vi "SRS865A--read--V2.vi"(8 "error in (no error)":errorcluster, 11 "VISA resource name":refnum<visa-resource-name>) -> (0 "error out":errorcluster, 1 "freq out":dbl, 2 "zi out (V)":cdb, 3 "VISA resource name out":refnum<visa-resource-name>)   [LabVIEW 2018]
uses:
  <instrlib>/Stanford Research SR865/Stanford Research SR865.lvlib
panel:
  out "read buffer 3":string
  out "read buffer 2":string
  out "read buffer":string
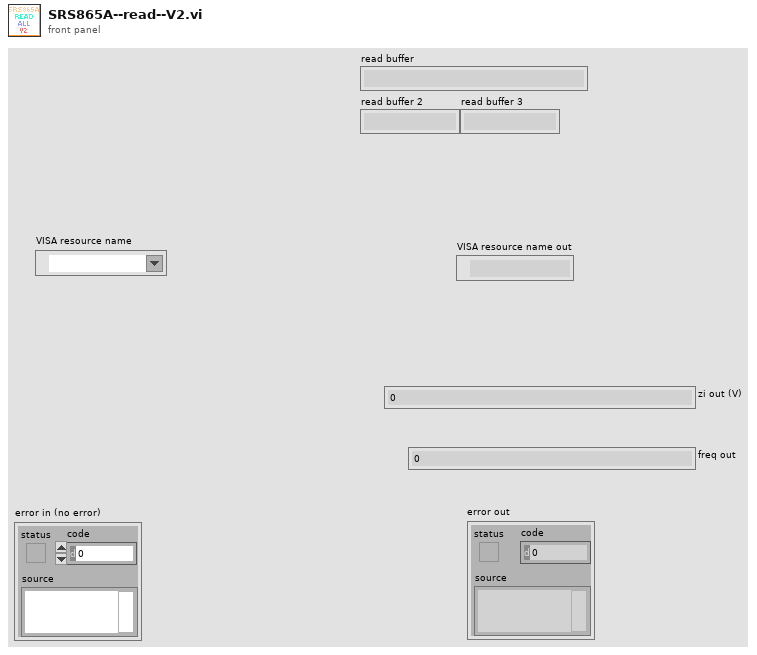
[diagram p1: front panel]
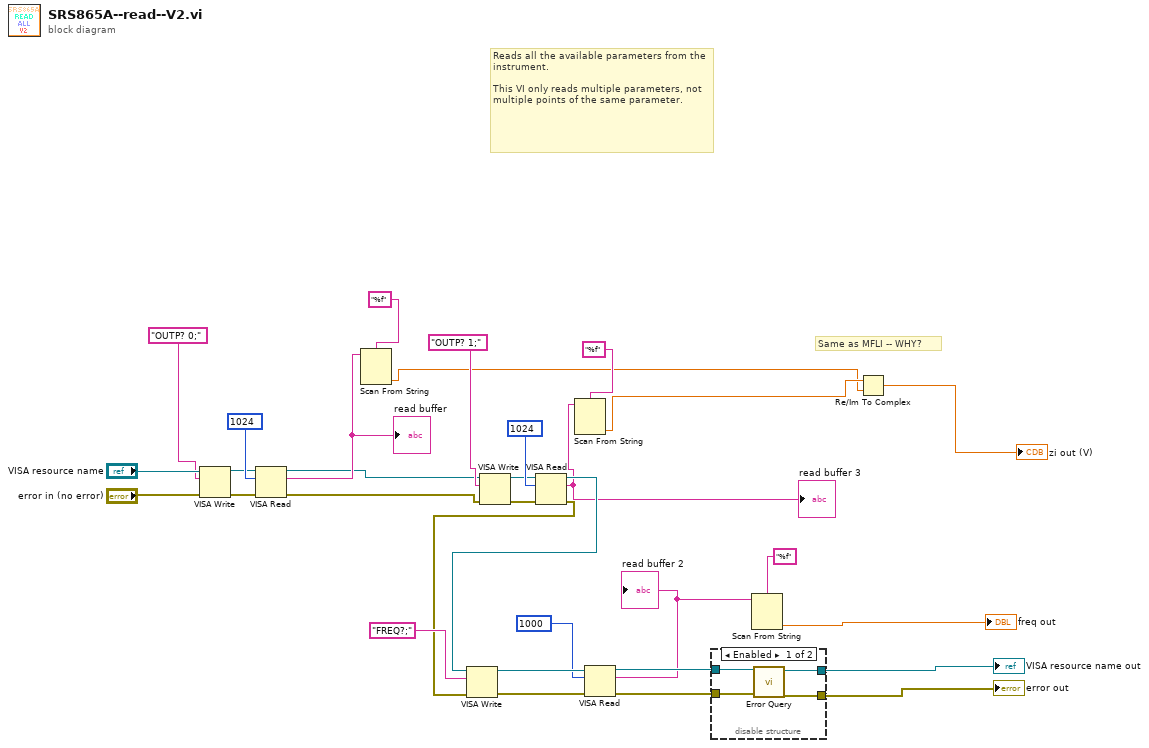
[diagram p0: block diagram]
diagram:
  # "Same as MFLI -- WHY?"
  # "Reads all the available parameters from the instrument.\n\nThis VI only reads multiple parameters, not multiple points of the same parameter."
  n1 = VISA Write(VISA resource name="VISA resource name", write buffer="OUTP? 0;", error in (no error)="error in (no error)") -> (VISA resource name out=w14:refnum<visa-resource-name>, error out=w31:errorcluster)  [unwired: 1 out]
  n2 = VISA Read(VISA resource name=w14, byte count=u32 1024, error in (no error)=w31) -> (VISA resource name out=w8:refnum<visa-resource-name>, read buffer=w27:string, error out=w6:errorcluster)  [unwired: 1 out]
  "read buffer" <- w27
  n3 = Scan From String(format string="%f", input string=w27) -> (output 1=w1:dbl)  [unwired: 3 in, 3 out]
  n4 = VISA Write(VISA resource name=w8, write buffer="OUTP? 1;", error in (no error)=w6) -> (VISA resource name out=w10:refnum<visa-resource-name>, error out=w12:errorcluster)  [unwired: 1 out]
  n5 = VISA Read(VISA resource name=w10, byte count=u32 1024, error in (no error)=w12) -> (VISA resource name out=w7:refnum<visa-resource-name>, read buffer=w3:string, error out=w5:errorcluster)  [unwired: 1 out]
  "read buffer 3" <- w3
  n6 = VISA Write(VISA resource name=w7, write buffer="FREQ?;", error in (no error)=w5) -> (VISA resource name out=w24:refnum<visa-resource-name>, error out=w22:errorcluster)  [unwired: 1 out]
  n7 = Scan From String(format string="%f", input string=w3) -> (output 1=w2:dbl)  [unwired: 3 in, 3 out]
  n8 = VISA Read(VISA resource name=w24, byte count=u32 1000, error in (no error)=w22) -> (VISA resource name out=w23:refnum<visa-resource-name>, read buffer=w20:string, error out=w21:errorcluster)  [unwired: 1 out]
  "read buffer 2" <- w20
  n9 = disable-structure shown="Enabled" {
    disable-tunnel: [w36 w38] -> w18
    disable-tunnel: [w35 w37] -> w17
    disable-tunnel: w23 -> [w34 w38]
    disable-tunnel: w21 -> [w33 w37]
    frame Enabled {
      n10 = call <instrlib>:"Error Query.vi"("error in (no error)"=w33, "VISA resource name"=w34) -> ("error out"=w35:errorcluster, "VISA resource name out"=w36:refnum<visa-resource-name>)  [unwired: 7 in, 1 out]
    }
    frame Disabled {
    }
  }
  "VISA resource name out" <- w18
  "error out" <- w17
  n11 = Scan From String(format string="%f", input string=w20) -> (output 1=→"freq out":dbl)  [unwired: 3 in, 3 out]
  n12 = Re/Im To Complex(1:w1, 2:w2) -> (0:→"zi out (V)":cdb)
